vi "INTELLIFAUCET Linear Interpolation GPMtouA.vi"(8 "Error In":errorcluster, 10 "Target":dbl, 11 "Interpolation Table(Xs,Ys)":dbl[][](array[numeric])=[[23.0, 6000.0], [37.0, 8400.0]]) -> (0 "Error Out":errorcluster, 2 "uA Output":i32)   [LabVIEW 2023]
uses:
  <vilib>/gmath/NI_Gmath.lvlib
panel:
  # "Need to add calibration file to fine tune this. Will make responcse better on the PID....or build conversion sheet during first purge"
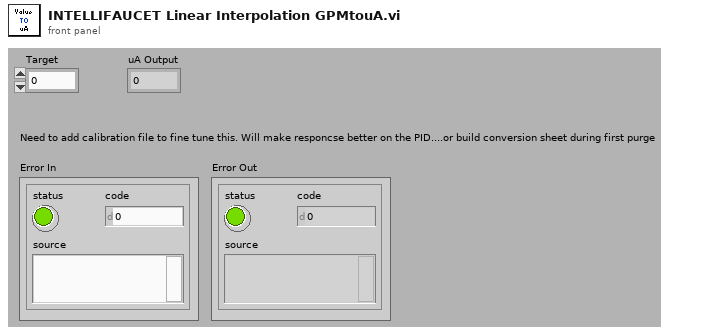
[diagram p1: front panel]
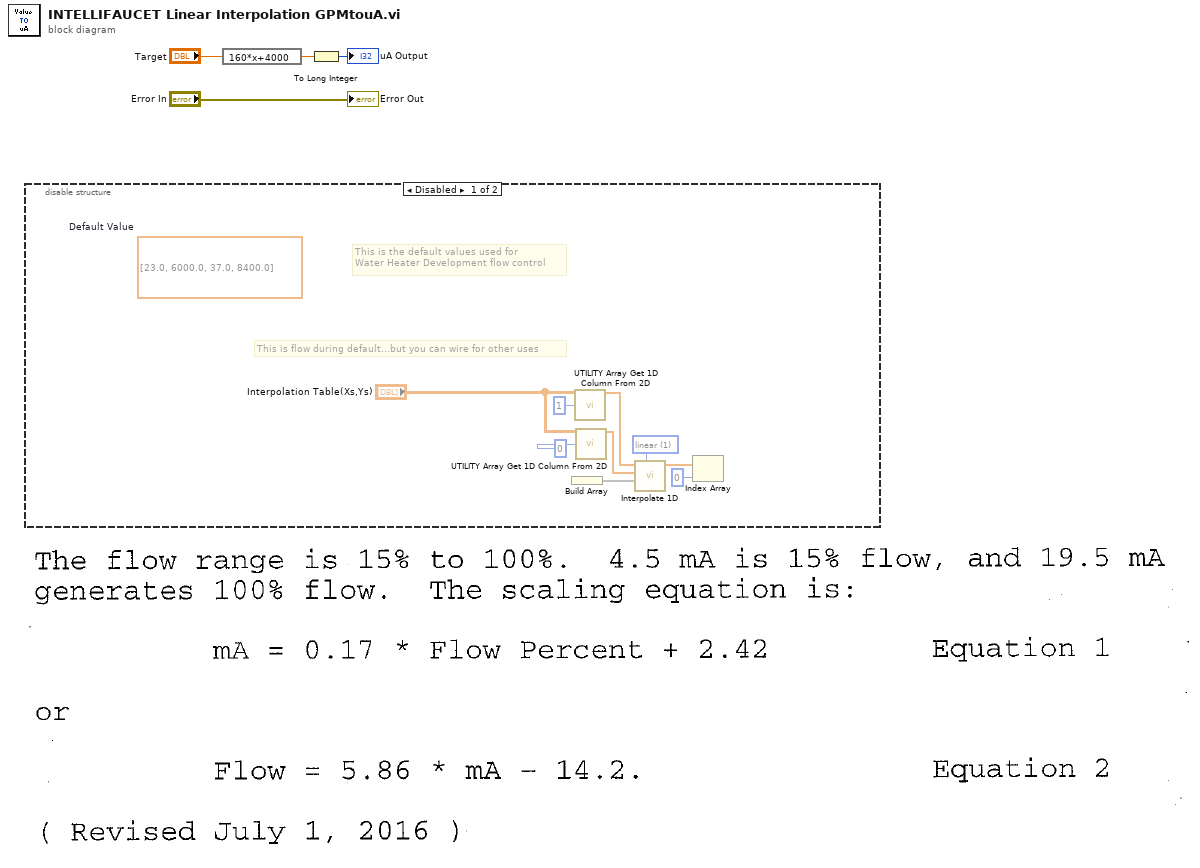
[diagram p0: block diagram]
diagram:
  n1 = disable-structure shown="Disabled" {
    frame Disabled {
      w5 = 1 items=["nearest", "linear", "spline", "cubic Hermite", "Lagrange"] ("method")
      (unwired) dbl[][] [[23.0, 6000.0], [37.0, 8400.0]]  # Default Value
      # "This is flow during default...but you can wire for other uses"
      # "This is the default values used for \nWater Heater Development flow control"
      n2 = Build Array() -> (w9:void[])  [unwired: 1 in]
      n3 = call "UTILITY Array Get 1D Column From 2D.vi"("2D Array Data"="Interpolation Table(Xs,Ys)", "column index"=1) -> ("Column Data"=w12:dbl[])  [unwired: 13 in]
      n4 = call "UTILITY Array Get 1D Column From 2D.vi"("2D Array Data"="Interpolation Table(Xs,Ys)", "column index"=0) -> ("Column Data"=w11:dbl[])  [unwired: 13 in]
      n5 = call <vilib>:"Interpolate 1D.vi"("method"=w5, "xi"=w9, "X"=w11, "Y"=w12) -> ("yi"=w10:dbl[])  [unwired: 5 in, 2 out]
      n6 = Index Array(array=w10, index=0) -> (element=w14:dbl)
    }
    frame Enabled {
    }
  }
  n7 = expression code="160*x+4000"("Target") -> (w2:dbl)
  n8 = To Long Integer(number=w2) -> (32bit integer=→"uA Output":i32)
  "Error Out" <- "Error In"
